vi "Sensor_Calidad_Aire.vi"(0 "COM Bluegiga in":refnum<visa-resource-name>, 3 "error in (no error)":errorcluster) -> (7 "COM Bluegiga out":refnum<visa-resource-name>, 8 "eCO2 ppm":dbl, 9 "TVOC ppb":dbl, 10 "error out":errorcluster)   [LabVIEW 2020]
panel:
  out "characteristic value":u8[](array[numeric])
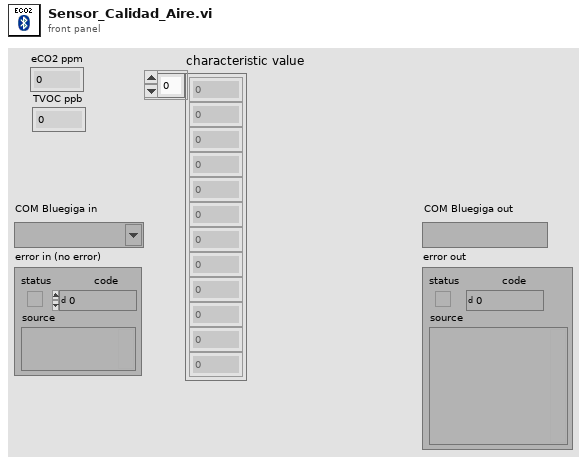
[diagram p1: front panel]
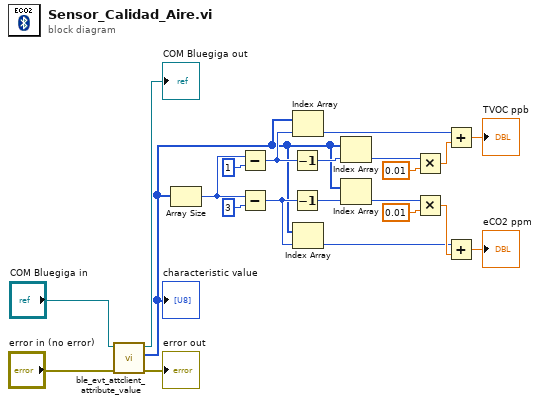
[diagram p0: block diagram]
diagram:
  n1 = call <vilib>:"ble_evt_attclient_attribute_value.vi"("error in (no error)"="error in (no error)", "COM Bluegiga in"="COM Bluegiga in") -> ("error out"=→"error out":errorcluster, "characteristic value"=w1:u8[], "COM Bluegiga out"=→"COM Bluegiga out":refnum<visa-resource-name>)  [unwired: 6 in, 1 out]
  "characteristic value" <- w1
  n2 = Array Size(array=w1) -> (size(s)=w5:i32)
  n3 = Subtract(x=w5, y=1) -> (x-y=w13:i32)
  n4 = Subtract(x=w5, y=3) -> (x-y=w6:i32)
  n5 = Decrement(x=w13) -> (x-1=w17:i32)
  n6 = Decrement(x=w6) -> (x-1=w11:i32)
  n7 = Index Array(array=w1, index=w13) -> (element=w2:u8)
  n8 = Index Array(array=w1, index=w6) -> (element=w7:u8)
  n9 = Index Array(array=w1, index=w17) -> (element=w16:u8)
  n10 = Index Array(array=w1, index=w11) -> (element=w10:u8)
  n11 = Multiply(x=w16, y=0.01) -> (x*y=w14:dbl)
  n12 = Multiply(x=w10, y=0.01) -> (x*y=w8:dbl)
  n13 = Add(x=w2, y=w14) -> (x+y=→"TVOC ppb":dbl)
  n14 = Add(x=w7, y=w8) -> (x+y=→"eCO2 ppm":dbl)
